vi "initialize s4ics.vi"(8 "error in (no error)":errorcluster, 11 "S4GEI in":refnum<class "S4GEI.lvclass">) -> (0 "error out":errorcluster, 3 "S4GEI out":refnum<class "S4GEI.lvclass">)   [LabVIEW 2018, in "S4GEI.lvclass"]
uses:
  S4GEI.lvclass
  S4GEI.lvclass/S4GEI.ctl
  S4ICS/S4ICS.lvclass
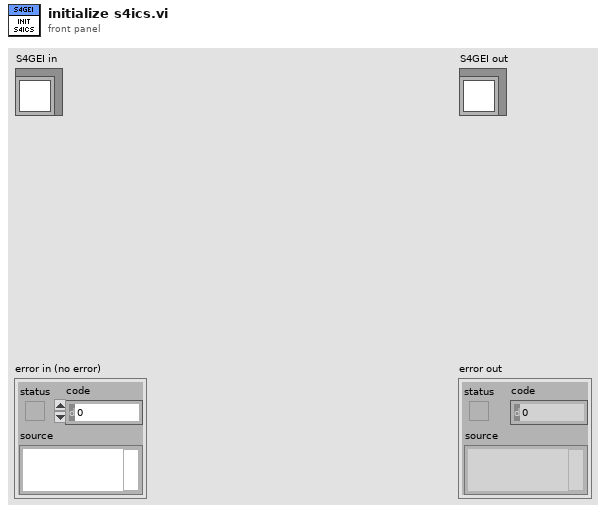
[diagram p1: front panel]
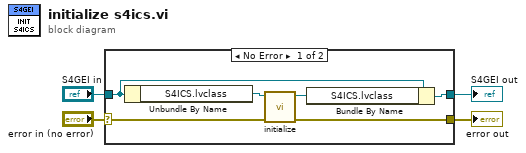
[diagram p0: block diagram]
diagram:
  n1 = case shown="No Error" "error in (no error)" {
    selector: "error in (no error)" -> [w7 w12]
    tunnel: [w5 w12] -> w3
    tunnel: [w9 w11] -> w1
    tunnel: "S4GEI in" -> [w10 w11]
    frame No Error {
      n2 = Unbundle By Name(w10) -> ("S4ICS.lvclass"=w8:refnum<class "S4ICS.lvclass">)
      n3 = call "initialize.vi"("error in (no error)"=w7, "S4ICS in"=w8) -> ("error out"=w5:errorcluster, "S4ICS out"=w6:refnum<class "S4ICS.lvclass">)  [unwired: 8 in]
      n4 = Bundle By Name(cluster=w10, "S4ICS.lvclass"=w6) -> (w9:refnum<class "S4GEI.lvclass">)
    }
    frame Error {
    }
  }
  "error out" <- w3
  "S4GEI out" <- w1
